vi "DAQ_PW_Check_time_out_to_turn_to_charging.vi"(8 "error in (no error)":errorcluster, 10 "USB_DEV_Json in":string, 11 "CT1_in":timestamp) -> (0 "error in (no error) 2":errorcluster, 2 "USB_DEV_Json out":string, 3 "CT1_out":timestamp)   [LabVIEW 2015]
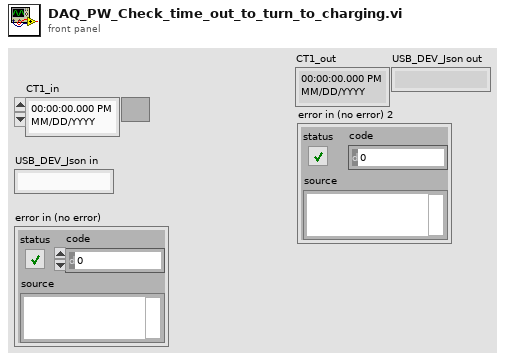
[diagram p1: front panel]
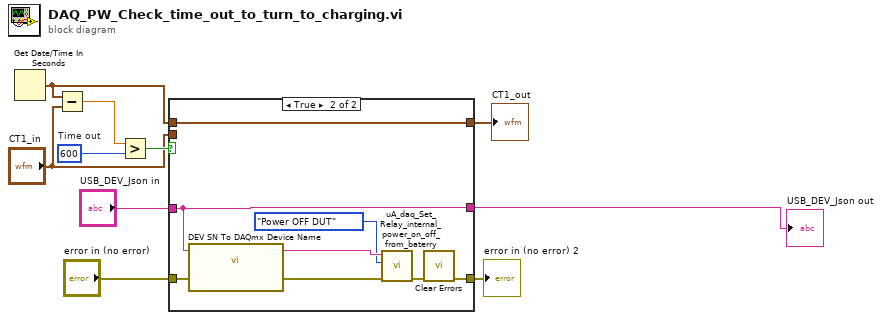
[diagram p0: block diagram]
diagram:
  w7 = u32 600  # Time out
  n1 = Get Date/Time In Seconds() -> (seconds since 1Jan1904=w3:timestamp)
  n2 = Subtract(x=w3, y="CT1_in") -> (x-y=w6:dbl)
  n3 = Greater?(x=w6, y=w7) -> (0:w8:bool)
  n4 = case shown="True" w8 {
    tunnel: "USB_DEV_Json in" -> [w11 w14]
    tunnel: "error in (no error)" -> [w12 w17]
    tunnel: "CT1_in" -> [w13 _]
    tunnel: [w13 w16] -> w4
    tunnel: w3 -> [_ w16]
    tunnel: [w12 w15] -> w2
    tunnel: [w11 w14] -> w1
    frame False {
    }
    frame True {
      n5 = call "DEV SN To DAQmx Device Name.vi"("error in (no error)"=w17, "USN_DEV (JSON)"=w14) -> ("error out"=w18:errorcluster, "DAQmx Device Name"=w21:tag)  [unwired: 8 in]
      n6 = call "uA_daq_Set_Relay_internal_power_on_off_from_baterry.vi"("error in"=w18, "Power ON/OFF DUT"=enum16{"Power ON DUT", "Power OFF DUT"}."Power OFF DUT", "USB DAQ"=w21) -> ("error out"=w19:errorcluster)  [unwired: 8 in]
      n7 = call <vilib>:"Clear Errors.vi"("error in (no error)"=w19) -> ("error out"=w15:errorcluster)  [unwired: 5 in, 1 out]
    }
  }
  "CT1_out" <- w4
  "error in (no error) 2" <- w2
  "USB_DEV_Json out" <- w1
